vi "titleAppend.vi"(10 "Final Title":string, 11 "String in":string) -> (3 "String out":string)   [LabVIEW 2012]
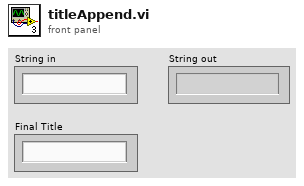
[diagram p1: front panel]
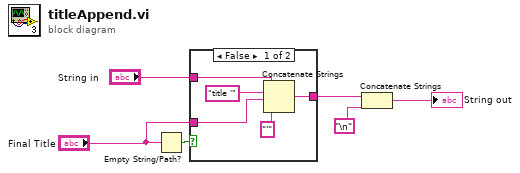
[diagram p0: block diagram]
diagram:
  n1 = Empty String/Path?(string/path="Final Title") -> (empty?=w3:bool)
  n2 = case shown="False" w3 {
    tunnel: "String in" -> [w11 w12]
    tunnel: [w9 w12] -> w5
    tunnel: "Final Title" -> [w7 _]
    frame False {
      n3 = Concatenate Strings(w11, "title '", w7, "'" ("string")) -> (w9:string)
    }
    frame True {
    }
  }
  n4 = Concatenate Strings(w5, "\n") -> (→"String out":string)
